vi "PADMINI_ ST1_REPORT.vi"(11 "String":string) -> (3 "appended array":string[](array[string]))   [LabVIEW 2017]
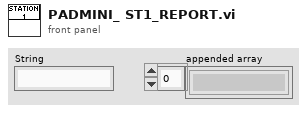
[diagram p1: front panel]
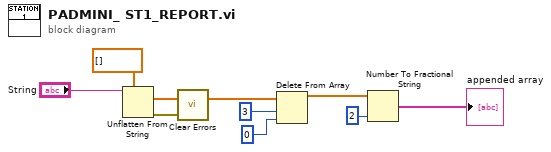
[diagram p0: block diagram]
diagram:
  n1 = Unflatten From String(type=dbl[] [] ("subarray"), binary string="String") -> (value=w6:dbl[], error out=w8:errorcluster)  [unwired: 3 in, 1 out]
  n2 = call <vilib>:"Clear Errors.vi"("error in (no error)"=w8) -> ()  [unwired: 5 in, 2 out]
  n3 = Delete From Array(array=w6, length=3, index=0) -> (array with subset deleted=w3:dbl[])  [unwired: 1 out]
  n4 = Number To Fractional String(number=w3, precision (6)=i16 2) -> (F-format string=→"appended array":string[])  [unwired: 2 in]
